vi "Parse (Internal Device Temperature).vi"(7 "Message In":string) -> (6 "Temperature":sgl, 15 "Timer":u32)   [LabVIEW 2012, in "MicroStrain 3DM-GXx.lvlib"]
doc: "Parse the data from the 0xD1 message into the device's internal temperature in degrees C."
uses:
  <instrlib>/MicroStrain 3DM-GXx/MicroStrain 3DM-GXx.lvlib
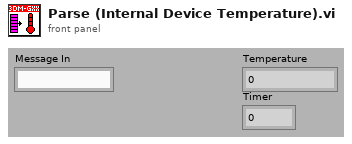
[diagram p1: front panel]
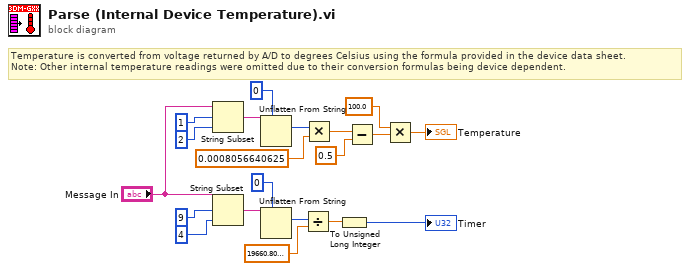
[diagram p0: block diagram]
diagram:
  # "Temperature is converted from voltage returned by A/D to degrees Celsius using the formula provided in the device data sheet.\nNote: Other internal temperature readings were omitted due to their conversion formulas being device dependent."
  n1 = String Subset(string="Message In", offset (0)=1, length (rest)=2 ("length (rest)")) -> (substring=w18:string)
  n2 = String Subset(string="Message In", offset (0)=9, length (rest)=4 ("length (rest)")) -> (substring=w13:string)
  n3 = Unflatten From String(type=u16 0, binary string=w18) -> (value=w1:u16)  [unwired: 3 in, 2 out]
  n4 = Unflatten From String(type=u32 0, binary string=w13) -> (value=w12:u32)  [unwired: 3 in, 2 out]
  n5 = Divide(x=w12, y=sgl 19660.8) -> (x/y=w10:sgl)
  n6 = Multiply(x=w1, y=0.0008056640625 ("x")) -> (x*y=w7:dbl)
  n7 = To Unsigned Long Integer(number=w10) -> (unsigned 32bit integer=→"Timer":u32)
  n8 = Subtract(x=w7, y=0.5) -> (x-y=w5:dbl)
  n9 = Multiply(x=100.0, y=w5) -> (x*y=→"Temperature":dbl)
